vi "Convert Hex String to String.vi"(11 "Hex String":string) -> (3 "String":string)   [LabVIEW 2020, in "MacroAssert.lvlib"]
doc: "Converts <B>Hex String</B> to a normal string."
uses:
  MacroAssert.lvlib
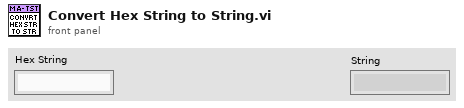
[diagram p1: front panel]
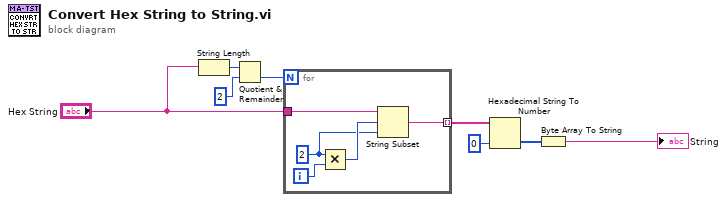
[diagram p0: block diagram]
diagram:
  n1 = String Length(string="Hex String") -> (length=w7:i32)
  n2 = Quotient & Remainder(x=w7, y=2) -> (floor(x/y)=w5:i32)  [unwired: 1 out]
  n3 = for {
    N: w5 -> [_]
    tunnel: "Hex String" -> [w13]
    tunnel: [w9] -> w4 mode=indexing
    i -> [w12]
    w10 = 2 ("x")
    n4 = Multiply(x=w10, y=w12) -> (x*y=w11:i32)
    n5 = String Subset(string=w13, offset (0)=w11, length (rest)=w10) -> (substring=w9:string)
  }
  n6 = Hexadecimal String To Number(string=w4, default (0uL)=u8 0 ("default (0 U32)")) -> (number=w3:u8[])  [unwired: 1 in, 1 out]
  n7 = Byte Array To String(unsigned byte array=w3) -> (string=→"String":string)
